vi "outputs.vi"() -> ()   [LabVIEW 2020]
doc: "This global variable contains current robot state information and actuator setpoints."
panel:
  out "Current_Driver_Profile_Setpoints":dbl[](array[numeric])
  out "LED_Colors":u32[](array[colorbox])
  out "LimeLight_LED_Mode":enum16{"Pipeline Setting", "Off", "Blink", "On"}(ring)=enum."Off"
  out "LimeLight_Pipeline":T1(ring)
  out "Force_Low_Gear":bool
  out "Swerve_2_High_Gear_Requested":bool
  out "Swerve_1_High_Gear_Requested":bool
  out "Swerve_3_High_Gear_Requested":bool
  out "Swerve_0_High_Gear_Requested":bool
  out "Swerve_2_Drive_Flip":bool
  out "Swerve_1_Drive_Flip":bool
  out "Swerve_3_Drive_Flip":bool
  out "Swerve_0_Drive_Flip":bool
  out "Swerve_3_Azimuth_Goal (deg)":dbl
  out "Swerve_1_Azimuth_Goal (deg)":dbl
  out "Swerve_2_Azimuth_Goal (deg)":dbl
  out "Swerve_0_Azimuth_Goal (deg)":dbl
  out "Diverting_Power_LEDS":bool
  out "Swerve_Rotation_Command":dbl
  out "Disallowed_Master_States":bool[](array[boolean])
  out "Drive_Mode":enum16{"Driver Control", "Lock Heading"}(ring)
  out "Diverting_Power_Compressor":bool
  out "Field_Oriented":bool
  out "Confirmed_Master_States":bool[](array[boolean])
  out "Boost_Drive_Current_Limit":bool
  out "Swerve_3_Azimuth_Error (deg)":dbl
  out "Swerve_1_Azimuth_Error (deg)":dbl
  out "Swerve_2_Azimuth_Error (deg)":dbl
  out "Swerve_0_Azimuth_Error (deg)":dbl
  out "Swerve_3_Drive_Command":dbl
  out "Swerve_1_Drive_Command":dbl
  out "Swerve_2_Drive_Command":dbl
  out "Swerve_0_Drive_Command":dbl
  # "--master state controller--"
  # "--drivebase subsystem--"
  # "--ball handling subsystem--"
  # "--power management--"
  # "--LL control--"
  # "--LEDs--"
  # "--climber subsystem--"
  # "--shooter subsystem--"
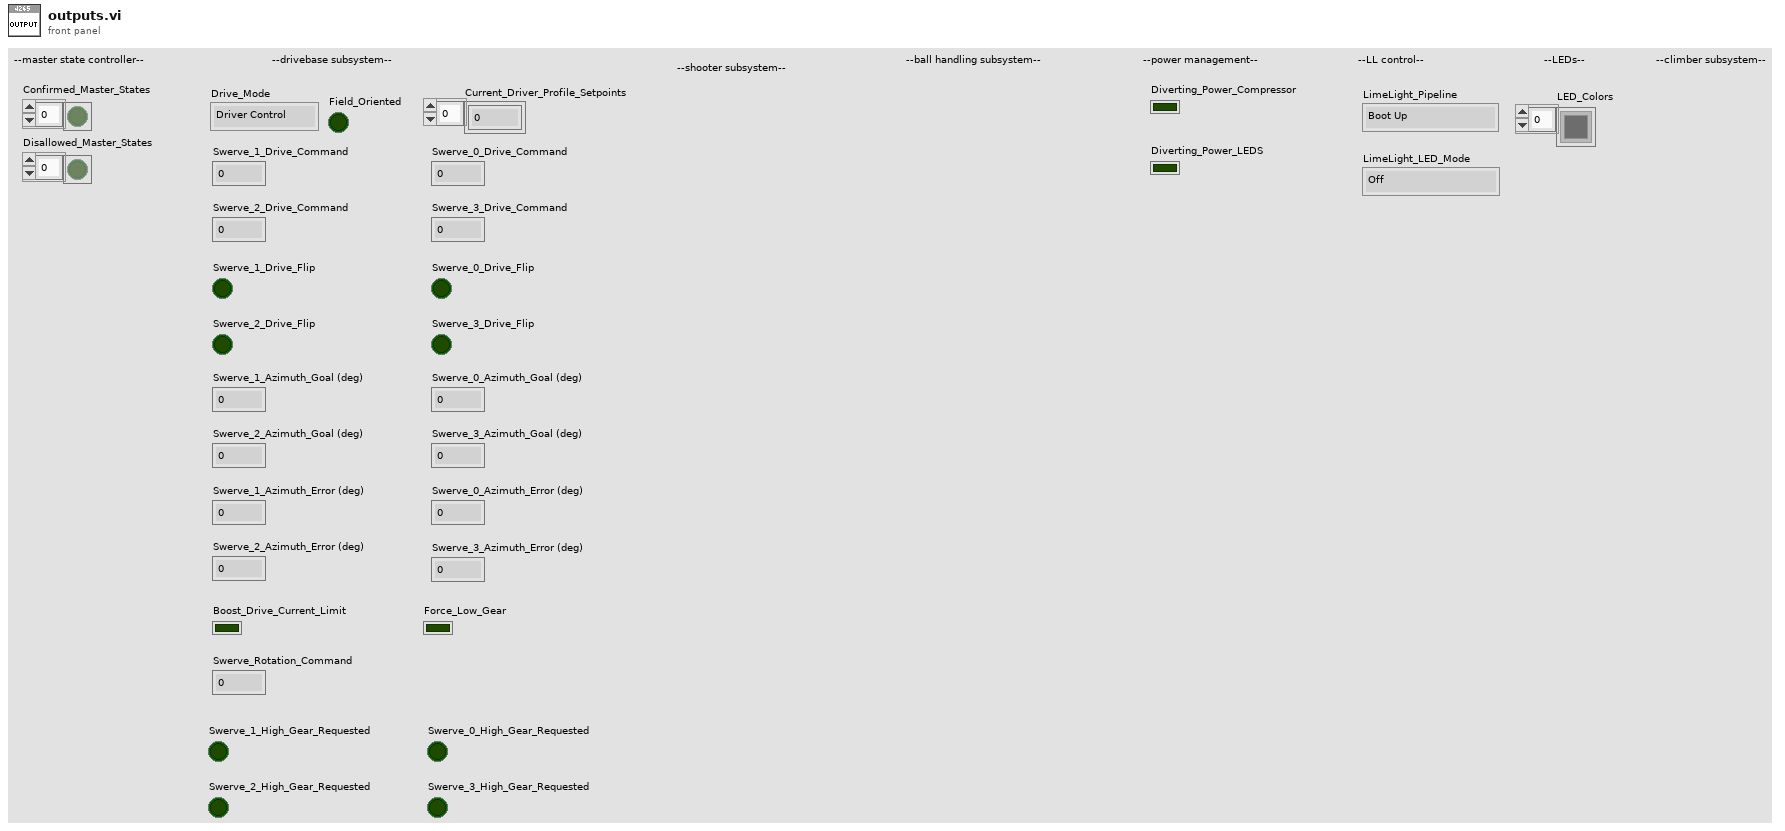
[diagram p1: front panel]
types:
  T1 = enum16{"Boot Up", "Camera Override", "Power Port", "Ball Tracking"}
diagram:
